vi "FindAllMessages.vi"(8 "error in (no error)":errorcluster, 11 "CS++Actor in":refnum<class "CS++Actor.lvclass">) -> (0 "error out":errorcluster, 3 "CS++Actor out":refnum<class "CS++Actor.lvclass">)   [LabVIEW 2014, in "CS++Actor.lvlib" / "CS++Actor.lvclass"]
doc: "Searches for all messages in this actor."
uses:
  CS++Actor.lvclass
  CS++Actor.lvclass/CS++Actor.ctl
  CSPP_Message/CS++Message.lvclass
  CSPP_Message/CS++Message.lvclass/CS++Message.ctl
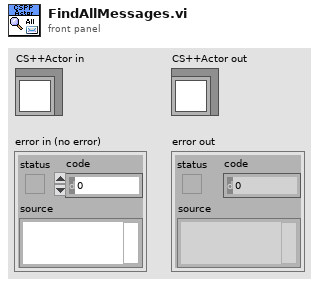
[diagram p1: front panel]
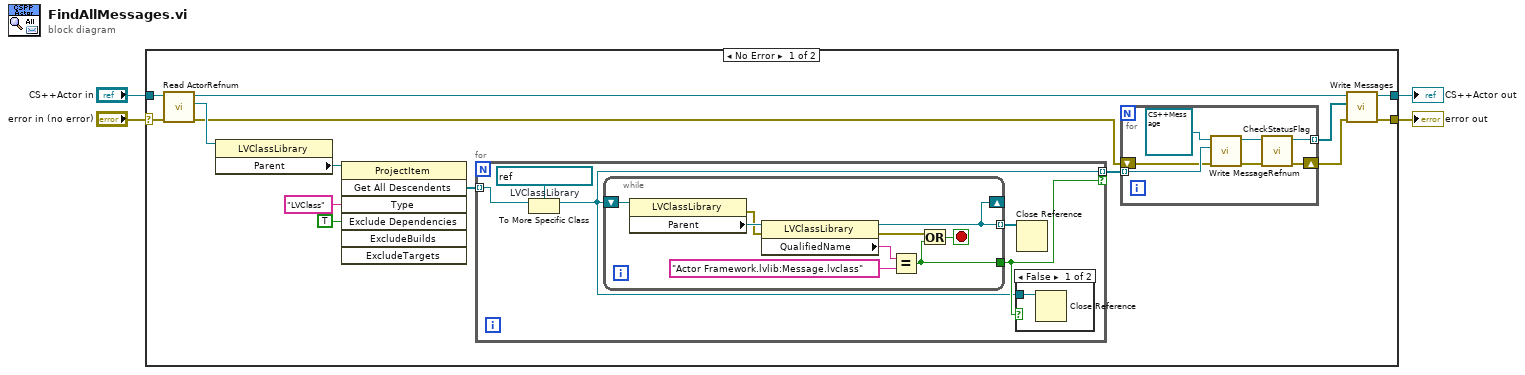
[diagram p0: block diagram]
diagram:
  n1 = case shown="No Error" "error in (no error)" {
    selector: "error in (no error)" -> [w13 w42]
    tunnel: [w8 w42] -> w3
    tunnel: [w6 w41] -> w1
    tunnel: "CS++Actor in" -> [w14 w41]
    frame No Error {
      n2 = call "Read ActorRefnum.vi"("error in (no error)"=w13, "CS++Actor in"=w14) -> ("error out"=w9:errorcluster, "ActorRefnum"=w12:refnum<vi>, "CS++Actor out"=w7:refnum<class "CS++Actor.lvclass">)  [unwired: 7 in]
      n3 = property class="LVClassLibrary"(reference=w12) -> ("Parent"=w16:refnum<vi>)  [unwired: 1 in, 2 out]
      n4 = invoke class="ProjectItem" method="Get All Descendents"(reference=w16, "Type"="LVClass", "Exclude Dependencies"=TRUE ("ExcludeDependencies")) -> ("All Descendents"=w15:refnum<vi>[])  [unwired: 4 in, 6 out]
      n5 = for {
        tunnel: w15 -> [w29] mode=indexing
        tunnel: [w26] -> w11 mode=indexing if=w27
        w30 = refnum<vi> refnum  # LVClassLibrary
        n6 = To More Specific Class(target class=w30, reference=w29) -> (specific class reference=w26:refnum<vi>)  [unwired: 1 in, 1 out]
        n7 = while {
          shift-right: [w34] -> _
          shift-left: w26 -> [w40]
          tunnel: [w34] -> w28 mode=indexing
          tunnel: [w33] -> w27
          stop <- w35 stop-if-true
          n8 = property class="LVClassLibrary"(reference=w40) -> (error out=w32:errorcluster, "Parent"=w36:refnum<vi>)  [unwired: 1 in, 1 out]
          n9 = property class="LVClassLibrary"(reference=w36, error in=w32) -> (reference out=w34:refnum<vi>, error out=w37:errorcluster, "QualifiedName"=w39:string)
          n10 = Equal?(x=w39, y="Actor Framework.lvlib:Message.lvclass") -> (x = y?=w33:bool)
          n11 = Or(x=w37, y=w33) -> (x .or. y?=w35:bool)
        }
        n12 = case shown="False" w27 {
          tunnel: w26 -> [w31 _]
          frame False {
            n13 = Close Reference(reference=w31) -> ()  [unwired: 1 in, 1 out]
          }
          frame True {
          }
        }
        n14 = Close Reference(reference=w28) -> ()  [unwired: 1 in, 1 out]
      }
      n15 = for {
        shift-right: [w19] -> w10
        shift-left: w9 -> [w23]
        tunnel: w11 -> [w24] mode=indexing
        tunnel: [w20] -> w5 mode=indexing
        n16 = call "Write MessageRefnum.vi"("error in (no error)"=w23, "MessageRefnum"=w24, "CS++Message in"=refnum<class "CS++Message.lvclass"> refnum ("CS++Message.lvlib:CS++Message.lvclass")) -> ("error out"=w21:errorcluster, "CS++Message out"=w22:refnum<class "CS++Message.lvclass">)  [unwired: 7 in]
        n17 = call "CheckStatusFlag.vi"("error in (no error)"=w21, "CS++Message in"=w22) -> ("error out"=w19:errorcluster, "CS++Message out"=w20:refnum<class "CS++Message.lvclass">)  [unwired: 8 in]
      }
      n18 = call "Write Messages.vi"("error in (no error)"=w10, "Messages"=w5, "CS++Actor in"=w7) -> ("error out"=w8:errorcluster, "CS++Actor out"=w6:refnum<class "CS++Actor.lvclass">)  [unwired: 7 in]
    }
    frame Error {
    }
  }
  "error out" <- w3
  "CS++Actor out" <- w1
